vi "FTW-Expression-Construct.vi"(5 "Lexicon":string, 11 "error in":errorcluster) -> (4 "Expression":refnum<class "FTW-Expression.lvclass">, 15 "error out":errorcluster)   [LabVIEW 2015, in "FTW-Expression.lvclass"]
uses:
  FTW-Expression.lvclass
  FTW-Expression.lvclass/FTW-Expression.ctl
panel:
  # "Inputs"
  # "Outputs"
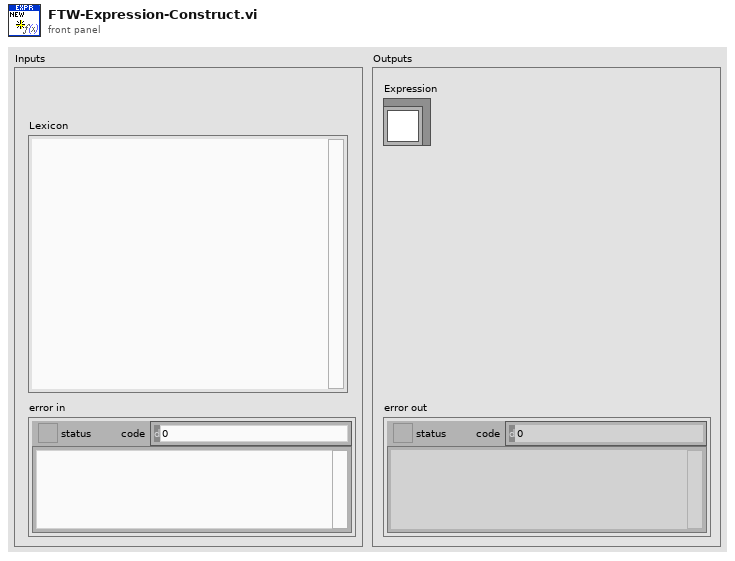
[diagram p1: front panel]
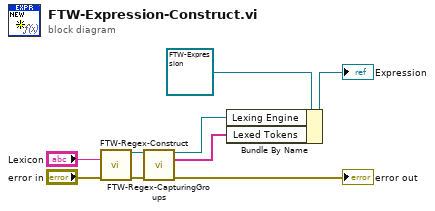
[diagram p0: block diagram]
diagram:
  n1 = call "FTW-Regex-Construct.vi"("Regular Expression"="Lexicon", "error in"="error in") -> ("Regex"=w9:refnum<data-value>, "error out"=w2:errorcluster)  [unwired: 12 in]
  n2 = call "FTW-Regex-CapturingGroups.vi"("Regex"=w9, "error in"=w2) -> ("Regex out"=w8:refnum<data-value>, "Capture Groups"=w7:string[], "error out"=→"error out":errorcluster)  [unwired: 11 in]
  n3 = Bundle By Name(cluster=refnum<class "FTW-Expression.lvclass"> refnum ("Expression"), "Lexing Engine"=w8, "Lexed Tokens"=w7) -> (→"Expression":refnum<class "FTW-Expression.lvclass">)
